vi "rxstop.vi"(8 "error in (no error)":errorcluster) -> (0 "rssi":i32, 1 "goodPackets":i32, 2 "crcErrPkt":i32, 3 "totalPkt":i32, 4 "error out":errorcluster)   [LabVIEW 2014]
uses:
  DLLTest.dll
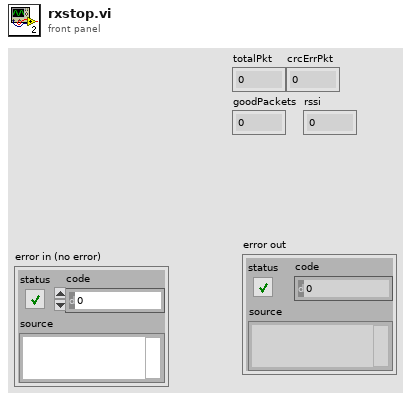
[diagram p1: front panel]
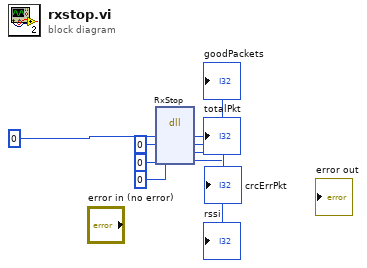
[diagram p0: block diagram]
diagram:
  n1 = dll-call lib="D:/Cobham_QCA9984/VI/DLLTest.dll" fn="RxStop"("totalPkt"=0, "goodPackets"=0, "crcErrPkt"=0, "rssi"=0) -> ("totalPkt"=→"totalPkt":i32, "goodPackets"=→"goodPackets":i32, "crcErrPkt"=→"crcErrPkt":i32, "rssi"=→"rssi":i32)  [unwired: 4 in, 2 out]
